vi "DOE Kitchen Agilent.vi"(1 "Flow Rate":dbl, 4 "Water Pressure":dbl, 5 "Data Logger Type":T13=enum."Agilent", 6 "Disable Digital":bool, 7 "Water Temperature":dbl, 8 "error in (no error)":errorcluster, 9 "Test Fixture Hardware":T7={"Power "={"Yokogawa"={"WT210"={"Sample Rate (1: 0.25s)"=1, "A Range (12: 20A)"=11, "V Range (6: 600V)"=4, "Power VISA Yokogawa WT210"=""}, "WT500"={"Power VISA Yokogawa WT500"="", "V Range (8: 1000V)"=6, "I Range (7: 40A)"=7, "Update Rate (3: 500ms)"=2}, "WT310_2"={"Sample Rate (1: 0.25s)"=1, "A Range (12: 20A)"=11, "V Range (6: 600V)"=4, "Power VISA Yokogawa WT310_2"=""}, "WT310_3"={"Sample Rate (1: 0.25s)"=1, "A Range (12: 20A)"=11, "V Range (6: 600V)"=4, "Power VISA Yokogawa WT310_3"=""}}, "Aplus"={"Aplus IP Address"="192.168.1.101", "Remote Port"=502, "Instrument"="APLUS", "Instr Driver Revision"="1.03.0053"}, "Power Limits"={"Crest Factor"={"Upper Limit"=1.49, "Lower Limit"=1.34}, "Harmonic Content"={"Uthd"=2.0}, "Voltage"={"% Error"=2.0}, "Stability"={"<1 Watt "={"Wattage"=1.0, "Slope (mW/H)"=10.0}, ">1 Watt"={"1%Power/Hour"=1.0}}}, "Nominal Voltage"=120, "Time Limit (s)"=10800.0, "Power Variation Limit (%)"=50.0, "Power Supply"={"Chroma 61605"="CHROMA", "Use Chroma?"=FALSE}}, "Weight Scale"={"Com Options"={"IND560Scale VISA"="MW100", "IP Address"="", "Remote Port"=502, "Setra Scale VISA"="MW100", "GSE 350"="GSE350"}, "Select Scale"=""}, "Flow Rates"={"Laurel Cold IP Address"="", "Laurel Hot IP Address"="", "Hot Water Laurel VISA"="LaurelMeter_Hot", "Cold Water Laurel VISA"="LaurelMeter_Cold", "Remote Port"=0, "Laurel Communication Type"="", "Meters To Collect (Hot Cold)"="", "HOT Laurel Reference"=refnum, "COLD Laurel Reference"=refnum}, "Analog Data"={"Agilent"={"Agilent 34972_1"="34972A_1", "Agilent 34972_2"="34972A_2", "Agilent 34972_3"="34972A_3", "Agilent 34972_4"="34972A_3", "Agilent 34972_5"="34972A_3", "Agilent 34972_6"="34972A_3", "Agilent Gain"=0.0, "TC Type (K,J,T)"="", "Instrument IDN?"="", "TC Channels-List"="", "Analog Channels-List"="", "Agilent Cluster Array"=[], "TC Channels-List 2"="", "Analog Channels-List 2"=""}, "Yokogawa"={"MW100"="MW100", "Intellifaucet"=FALSE}, "Select Analog"="", "TC Coefficients"={"TC Coefficients 1"=[], "TC Coefficients 2"=[], "TC Coefficients 3"=[], "TC Coefficients 4"=[], "TC Coefficients 5"=[], "TC Coefficients 6"=[], "TC Coefficients 7"=[]}, "NI Tasks (Dryer DOE)"=["TC Temps-Module 1", "TC Temps-Module 2", "TC Temps-Module 3", "TC Temps-Module 4", "TC Temps-Module 5", "Gas and Temp-Module 6", "AC_DC Events-Module 7"], "Laurel Analog"={"Laurel IP (Water Temp)"="", "Laurel IP (Pressure)"=""}}, "ITHX-Temp Humidity"={"IP Address 1"="", "Remote Port"=0, "IP Address 2"="", "IP Address 3"=""}, "Gas Meter COM Ports"={"Gas Meter 1"="COM3", "Gas Meter 2"="COM4", "Gas Meter 3"="COM5", "Gas Meter 4"="COM6", "Gas Meter 5"="COM7", "Gas Meter 6"="COM8"}, "Barometric Pressure"={"HEISE 901A"="HEISE", "Use Barometer?"=FALSE}} {"Power"."Yokogawa"."WT310_3"."V Range (6: 600V)" items=["Auto", "15V", "30V", "60V", "150V", "300V", "600V"]; "Power"."Yokogawa"."WT310_3"."A Range (12: 20A)" items=["Auto", "5mA", "10mA", "20mA", "50mA", "100mA", "200mA", "0.5A", "1A", "2A", "5A", "10A", "20A", "50mV", "100mV", "200mV", "2.5V", "5V", "10V"]; "Power"."Yokogawa"."WT310_3"."Sample Rate (1: 0.25s)" items=["0.1s", "0.25s", "0.5s", "1s", "2s", "5s"]; "Power"."Yokogawa"."WT310_2"."V Range (6: 600V)" items=["Auto", "15V", "30V", "60V", "150V", "300V", "600V"]; "Power"."Yokogawa"."WT310_2"."A Range (12: 20A)" items=["Auto", "5mA", "10mA", "20mA", "50mA", "100mA", "200mA", "0.5A", "1A", "2A", "5A", "10A", "20A", "50mV", "100mV", "200mV", "2.5V", "5V", "10V"]; "Power"."Yokogawa"."WT310_2"."Sample Rate (1: 0.25s)" items=["0.1s", "0.25s", "0.5s", "1s", "2s", "5s"]; "Power"."Yokogawa"."WT500"."Update Rate (3: 500ms)" items=["-", "100ms", "200ms", "500ms", "1s", "2s", "5s"]; "Power"."Yokogawa"."WT500"."I Range (7: 40A)" items=["AUTO", "500 mA", "1 A", "2 A", "5 A", "10 A", "20 A", "40 A", "S-AUTO", "50 mV", "100 mV", "200 mV", "500 mV", "1 V", "2 V", "5 V", "10 V", "250 mA", "500 mA", "1 A", "2.5 A", "5 A", "10 A", "20 A", "25 mV", "50 mV", "100 mV", "250 mV", "500 mV", "1 V", "2.5 V", "5 V"]; "Power"."Yokogawa"."WT500"."V Range (8: 1000V)" items=["AUTO", "15", "30", "60", "100", "150", "300", "600", "1000", "7.5", "15", "30", "50", "75", "150", "300", "500"]; "Power"."Yokogawa"."WT210"."V Range (6: 600V)" items=["Auto", "15V", "30V", "60V", "150V", "300V", "600V"]; "Power"."Yokogawa"."WT210"."A Range (12: 20A)" items=["Auto", "5mA", "10mA", "20mA", "50mA", "100mA", "200mA", "0.5A", "1A", "2A", "5A", "10A", "20A", "50mV", "100mV", "200mV", "2.5V", "5V", "10V"]; "Power"."Yokogawa"."WT210"."Sample Rate (1: 0.25s)" items=["0.1s", "0.25s", "0.5s", "1s", "2s", "5s"]}, 10 "Measurments":T1={"Power Measurements"={"Current (A):Element 1"=0.0, "Current (A):Element 2"=0.0, "Power (W):Sigma"=0.0, "Watt Hours (Wh):Sigma"=0.0, "Voltage (V):Element 2"=0.0, "Voltage (V):Element 1"=0.0, "Current Crest Factor:Element 1"=0.0, "Current Crest Factor:Element 2"=0.0, "Voltage Harmonic (%):Element 1"=0.0, "Voltage Harmonic (%):Element 2"=0.0, "Voltage Crest Factor:Element 1"=0.0, "Voltage Crest Factor:Element 2"=0.0, "Time:Element 1"=0.0, "Frequency (Hz):Element 1"=0.0, "Apparent Power (VA):Element 1"=0.0, "Apparent Power (VA):Element 2"=0.0, "Power Factor:Element 1"=0.0, "Power Factor:Element 2"=0.0, "Max Watt Hours"=0.0, "Voltage (V):Element 2 Avg"=0.0, "Voltage (V):Element 1 Avg"=0.0}, "Standby Power"={"Standby Power Spreadsheet"=[], "Standby Power - Pia (Watts)"=0.0, "Off Mode Power - Poff (Watts)"=0.0, "Sia hr/yr"=8620.0, "Soff hr/yr"=0.0, "Yearly Energy Etso kWh/yr"=0.0, "Maximum Power (Watts)"=0.0, "Power Variation (%)"=0.0, "Slope (mW/hr)"=0.0, "Final Harmonics-U1 (%)"="", "Final Harmonics-U2 (%)"="", "Energy (Wh)"=0.0}, "Washer"={"Washer String Data"=[], "Analog Scale Weight (lbs)"=0.0}, "Dishwasher"={"Drain Solonoid Event"=0, "Pump Event"=0, "Water Valve Event"=0, "Heater Event"=0, "Motor Event"=0, "Turbidity Sensor"=0.0, "Spare 2"=0.0, "Spare 3"=0.0, "Spare 4"=0.0, "Spare 5"=0.0, "Thermocouple 1"=0.0, "Thermocouple 2"=0.0, "Thermocouple 3"=0.0, "Thermocouple 4"=0.0, "Thermocouple 5"=0.0, "Thermocouple 6"=0.0, "Spare 1"=0.0, "Dishwasher String Data"=[]}, "Washer HCC"={"Chan 101"=0.0, "Chan 102"=0.0, "Chan 103"=0.0, "Chan 104"=0.0, "Chan 105"=0.0, "Chan 106"=0.0, "Chan 107"=0.0, "Chan 108"=0.0, "Chan 109"=0.0, "Chan 110"=0.0, "Chan 111"=0.0, "Chan 112"=0.0, "Chan 113"=0.0, "Chan 114"=0.0, "Chan 115"=0.0, "Chan 116"=0.0, "Chan 117"=0.0, "Chan 118"=0.0, "Chan 119"=0.0, "Chan 120"=0.0, "Chan 201"=0.0, "Chan 202"=0.0, "Chan 203"=0.0, "Chan 204"=0.0, "Chan 205"=0.0, "Chan 206"=0.0, "Chan 207"=0.0, "Chan 208"=0.0, "Chan 209"=0.0, "Chan 210"=0.0, "Chan 211"=0.0, "Chan 212"=0.0, "Chan 213"=0.0, "Chan 214"=0.0, "Chan 215"=0.0, "Chan 216"=0.0, "Chan 217"=0.0, "Chan 218"=0.0, "Chan 219"=0.0, "Chan 220"=0.0, "Chan 301"=0.0, "Chan 302"=0.0, "Chan 303"=0.0, "Chan 304"=0.0, "Chan 305"=0.0, "Chan 306"=0.0, "Chan 307"=0.0, "Chan 308"=0.0, "Chan 309"=0.0, "Chan 310"=0.0, "Chan 311"=0.0, "Chan 312"=0.0, "Chan 313"=0.0, "Chan 314"=0.0, "Chan 315"=0.0, "Chan 316"=0.0, "Chan 317"=0.0, "Chan 318"=0.0, "Chan 319"=0.0, "Chan 320"=0.0}, "Barometric Pressure"={"Barometric Pressure (in. Hg)"=0.0}, "Ambient Conditions"={"Ambient Temperature  1 (°F)"=0.0, "Ambient Temperature 2 (°F)"=0.0, "Ambient Temperature 3 (°F)"=0.0, "Ambient Humidity 1 (%)"=0.0, "Ambient Humidity 2 (%)"=0.0, "Ambient Humidity 3 (%)"=0.0, "Ambient Dewpoint  1 (°F)"=0.0, "Ambient Dewpoint 2 (°F)"=0.0, "Ambient Dewpoint 3 (°F)"=0.0}, "Weight Scale"={"Gross Weigth (lbs)"=0.0, "Net Weight (lbs)"=0.0, "Final Weight (lbs)"=""}, "Water Measurements"={"Hot Water Pressure (psi)"=0.0, "Hot Water Pressure Max (psi)"=0.0, "Hot Water Temperature (°F)"=0.0, "Cold Water Pressure (psi)"=0.0, "Cold Water Pressure Max (psi)"=0.0, "Hot Water Temperature Max (°F)"=0.0, "Cold Water Temperature (°F)"=0.0, "Cold Water Temperature Max (°F)"=0.0, "Hot Water Total (Gal)"=0.0, "Hot Water Rate (GPM)"=0.0, "Cold Water Total (Gal)"=0.0, "Cold Water Rate (GPM)"=0.0, "Cold Water Total During Wash (Gal)"=0.0, "Hot Water Total During Wash (Gal)"=0.0, "Rinse Cold (Gal)"=0.0, "Rinse Hot (Gal)"=0.0, "Hot Water Pressure Min (psi)"=0.0, "Hot Water Temperature Min (°F)"=0.0, "Cold Water Pressure Min (psi)"=0.0, "Cold Water Temperature Min (°F)"=0.0}, "Gas Data"={"Meter Type (Gas)"="", "Meter ID"=enum."Disabled", "Heating Value (BTU/ft³)"=0.0, "Ft³ / Hr (SCFH)"=0.0, "15 Second Average (BTU/HR)"=0.0, "30 Second Average (BTU/HR)"=0.0, "SLPM (Mass Flow)"=0.0, "LPM (Vol. Flow)"=0.0, "Gas Temperature (°F)"=0.0, "Gas Pressure (PSIA)"=0.0, "Tot.Flow (Liters)"=0.0}} {"Power Measurements"."Voltage (V):Element 1 Avg" format="%.3g"; "Power Measurements"."Voltage (V):Element 2 Avg" format="%.3g"; "Power Measurements"."Max Watt Hours" format="%.3g"; "Power Measurements"."Power Factor:Element 2" format="%.3g"; "Power Measurements"."Power Factor:Element 1" format="%.3g"; "Power Measurements"."Apparent Power (VA):Element 2" format="%.3g"; "Power Measurements"."Apparent Power (VA):Element 1" format="%.3g"; "Power Measurements"."Frequency (Hz):Element 1" format="%.3g"; "Power Measurements"."Time:Element 1" format="%.3g"; "Power Measurements"."Voltage Crest Factor:Element 2" format="%.3g"; "Power Measurements"."Voltage Crest Factor:Element 1" format="%.3g"; "Power Measurements"."Voltage Harmonic (%):Element 2" format="%.3g"; "Power Measurements"."Voltage Harmonic (%):Element 1" format="%.3g"; "Power Measurements"."Current Crest Factor:Element 2" format="%.3g"; "Power Measurements"."Current Crest Factor:Element 1" format="%.3g"; "Power Measurements"."Voltage (V):Element 1" format="%.3g"; "Power Measurements"."Voltage (V):Element 2" format="%.3g"; "Power Measurements"."Watt Hours (Wh):Sigma" format="%.3f"; "Power Measurements"."Power (W):Sigma" format="%.3g"; "Power Measurements"."Current (A):Element 2" format="%.3g"; "Power Measurements"."Current (A):Element 1" format="%.3g"}, 11 "VISA Resource Name":refnum<visa-resource-name>) -> (0 "error out":errorcluster, 2 "Measurments Output":T1={"Power Measurements"={"Current (A):Element 1"=0.0, "Current (A):Element 2"=0.0, "Power (W):Sigma"=0.0, "Watt Hours (Wh):Sigma"=0.0, "Voltage (V):Element 2"=0.0, "Voltage (V):Element 1"=0.0, "Current Crest Factor:Element 1"=0.0, "Current Crest Factor:Element 2"=0.0, "Voltage Harmonic (%):Element 1"=0.0, "Voltage Harmonic (%):Element 2"=0.0, "Voltage Crest Factor:Element 1"=0.0, "Voltage Crest Factor:Element 2"=0.0, "Time:Element 1"=0.0, "Frequency (Hz):Element 1"=0.0, "Apparent Power (VA):Element 1"=0.0, "Apparent Power (VA):Element 2"=0.0, "Power Factor:Element 1"=0.0, "Power Factor:Element 2"=0.0, "Max Watt Hours"=0.0, "Voltage (V):Element 2 Avg"=0.0, "Voltage (V):Element 1 Avg"=0.0}, "Standby Power"={"Standby Power Spreadsheet"=[], "Standby Power - Pia (Watts)"=0.0, "Off Mode Power - Poff (Watts)"=0.0, "Sia hr/yr"=8620.0, "Soff hr/yr"=0.0, "Yearly Energy Etso kWh/yr"=0.0, "Maximum Power (Watts)"=0.0, "Power Variation (%)"=0.0, "Slope (mW/hr)"=0.0, "Final Harmonics-U1 (%)"="", "Final Harmonics-U2 (%)"="", "Energy (Wh)"=0.0}, "Washer"={"Washer String Data"=[], "Analog Scale Weight (lbs)"=0.0}, "Dishwasher"={"Drain Solonoid Event"=0, "Pump Event"=0, "Water Valve Event"=0, "Heater Event"=0, "Motor Event"=0, "Turbidity Sensor"=0.0, "Spare 2"=0.0, "Spare 3"=0.0, "Spare 4"=0.0, "Spare 5"=0.0, "Thermocouple 1"=0.0, "Thermocouple 2"=0.0, "Thermocouple 3"=0.0, "Thermocouple 4"=0.0, "Thermocouple 5"=0.0, "Thermocouple 6"=0.0, "Spare 1"=0.0, "Dishwasher String Data"=[]}, "Washer HCC"={"Chan 101"=0.0, "Chan 102"=0.0, "Chan 103"=0.0, "Chan 104"=0.0, "Chan 105"=0.0, "Chan 106"=0.0, "Chan 107"=0.0, "Chan 108"=0.0, "Chan 109"=0.0, "Chan 110"=0.0, "Chan 111"=0.0, "Chan 112"=0.0, "Chan 113"=0.0, "Chan 114"=0.0, "Chan 115"=0.0, "Chan 116"=0.0, "Chan 117"=0.0, "Chan 118"=0.0, "Chan 119"=0.0, "Chan 120"=0.0, "Chan 201"=0.0, "Chan 202"=0.0, "Chan 203"=0.0, "Chan 204"=0.0, "Chan 205"=0.0, "Chan 206"=0.0, "Chan 207"=0.0, "Chan 208"=0.0, "Chan 209"=0.0, "Chan 210"=0.0, "Chan 211"=0.0, "Chan 212"=0.0, "Chan 213"=0.0, "Chan 214"=0.0, "Chan 215"=0.0, "Chan 216"=0.0, "Chan 217"=0.0, "Chan 218"=0.0, "Chan 219"=0.0, "Chan 220"=0.0, "Chan 301"=0.0, "Chan 302"=0.0, "Chan 303"=0.0, "Chan 304"=0.0, "Chan 305"=0.0, "Chan 306"=0.0, "Chan 307"=0.0, "Chan 308"=0.0, "Chan 309"=0.0, "Chan 310"=0.0, "Chan 311"=0.0, "Chan 312"=0.0, "Chan 313"=0.0, "Chan 314"=0.0, "Chan 315"=0.0, "Chan 316"=0.0, "Chan 317"=0.0, "Chan 318"=0.0, "Chan 319"=0.0, "Chan 320"=0.0}, "Barometric Pressure"={"Barometric Pressure (in. Hg)"=0.0}, "Ambient Conditions"={"Ambient Temperature  1 (°F)"=0.0, "Ambient Temperature 2 (°F)"=0.0, "Ambient Temperature 3 (°F)"=0.0, "Ambient Humidity 1 (%)"=0.0, "Ambient Humidity 2 (%)"=0.0, "Ambient Humidity 3 (%)"=0.0, "Ambient Dewpoint  1 (°F)"=0.0, "Ambient Dewpoint 2 (°F)"=0.0, "Ambient Dewpoint 3 (°F)"=0.0}, "Weight Scale"={"Gross Weigth (lbs)"=0.0, "Net Weight (lbs)"=0.0, "Final Weight (lbs)"=""}, "Water Measurements"={"Hot Water Pressure (psi)"=0.0, "Hot Water Pressure Max (psi)"=0.0, "Hot Water Temperature (°F)"=0.0, "Cold Water Pressure (psi)"=0.0, "Cold Water Pressure Max (psi)"=0.0, "Hot Water Temperature Max (°F)"=0.0, "Cold Water Temperature (°F)"=0.0, "Cold Water Temperature Max (°F)"=0.0, "Hot Water Total (Gal)"=0.0, "Hot Water Rate (GPM)"=0.0, "Cold Water Total (Gal)"=0.0, "Cold Water Rate (GPM)"=0.0, "Cold Water Total During Wash (Gal)"=0.0, "Hot Water Total During Wash (Gal)"=0.0, "Rinse Cold (Gal)"=0.0, "Rinse Hot (Gal)"=0.0, "Hot Water Pressure Min (psi)"=0.0, "Hot Water Temperature Min (°F)"=0.0, "Cold Water Pressure Min (psi)"=0.0, "Cold Water Temperature Min (°F)"=0.0}, "Gas Data"={"Meter Type (Gas)"="", "Meter ID"=enum."Disabled", "Heating Value (BTU/ft³)"=0.0, "Ft³ / Hr (SCFH)"=0.0, "15 Second Average (BTU/HR)"=0.0, "30 Second Average (BTU/HR)"=0.0, "SLPM (Mass Flow)"=0.0, "LPM (Vol. Flow)"=0.0, "Gas Temperature (°F)"=0.0, "Gas Pressure (PSIA)"=0.0, "Tot.Flow (Liters)"=0.0}} {"Power Measurements"."Voltage (V):Element 1 Avg" format="%.3g"; "Power Measurements"."Voltage (V):Element 2 Avg" format="%.3g"; "Power Measurements"."Max Watt Hours" format="%.3g"; "Power Measurements"."Power Factor:Element 2" format="%.3g"; "Power Measurements"."Power Factor:Element 1" format="%.3g"; "Power Measurements"."Apparent Power (VA):Element 2" format="%.3g"; "Power Measurements"."Apparent Power (VA):Element 1" format="%.3g"; "Power Measurements"."Frequency (Hz):Element 1" format="%.3g"; "Power Measurements"."Time:Element 1" format="%.3g"; "Power Measurements"."Voltage Crest Factor:Element 2" format="%.3g"; "Power Measurements"."Voltage Crest Factor:Element 1" format="%.3g"; "Power Measurements"."Voltage Harmonic (%):Element 2" format="%.3g"; "Power Measurements"."Voltage Harmonic (%):Element 1" format="%.3g"; "Power Measurements"."Current Crest Factor:Element 2" format="%.3g"; "Power Measurements"."Current Crest Factor:Element 1" format="%.3g"; "Power Measurements"."Voltage (V):Element 1" format="%.3g"; "Power Measurements"."Voltage (V):Element 2" format="%.3g"; "Power Measurements"."Watt Hours (Wh):Sigma" format="%.3f"; "Power Measurements"."Power (W):Sigma" format="%.3g"; "Power Measurements"."Current (A):Element 2" format="%.3g"; "Power Measurements"."Current (A):Element 1" format="%.3g"}, 3 "Kitchen Analog Data":string[][](array[string]))   [LabVIEW 2018]
uses:
  Type Definitions/DOE Data Logger Type.ctl
  Type Definitions/DOE Test Fixture Hardware.ctl
  Utility/Type Definitions/UTILITY Power Inputs Control.ctl
  Drivers/IND560 Scale Monitor/Type Definitions/IND560 Configuration.ctl
  Hybrid Water Heater/Type Definitions/HEWH Agilent Cluster.ctl
  Utility/Type Definitions/UTILITY TC Coefficients.ctl
  Drivers/Omega FMA-1600A Series Gas Flow Meter/Type Definitions/FMA1600A COM Ports.ctl
  Type Definitions/DOE Front Panel Meters.ctl
  Utility/Type Definitions/UTILITY Power Data.ctl
  Utility/Standby Power/Type Definitions/Standby Power Main Data.ctl
  Drivers/Omega FMA-1600A Series Gas Flow Meter/Type Definitions/FMA1600A Gas Data.ctl
  Drivers/Omega FMA-1600A Series Gas Flow Meter/Type Definitions/FMA1600A Gas Type.ctl
  Range/Type Definitions/RANGE Meter Selector 1-2.ctl
  Drivers/Yokogawa MW100/Type Definitions/YKMW100 DISH Channel Settings.ctl
  Drivers/Agilent 34972/Agilent 34970.lvlib
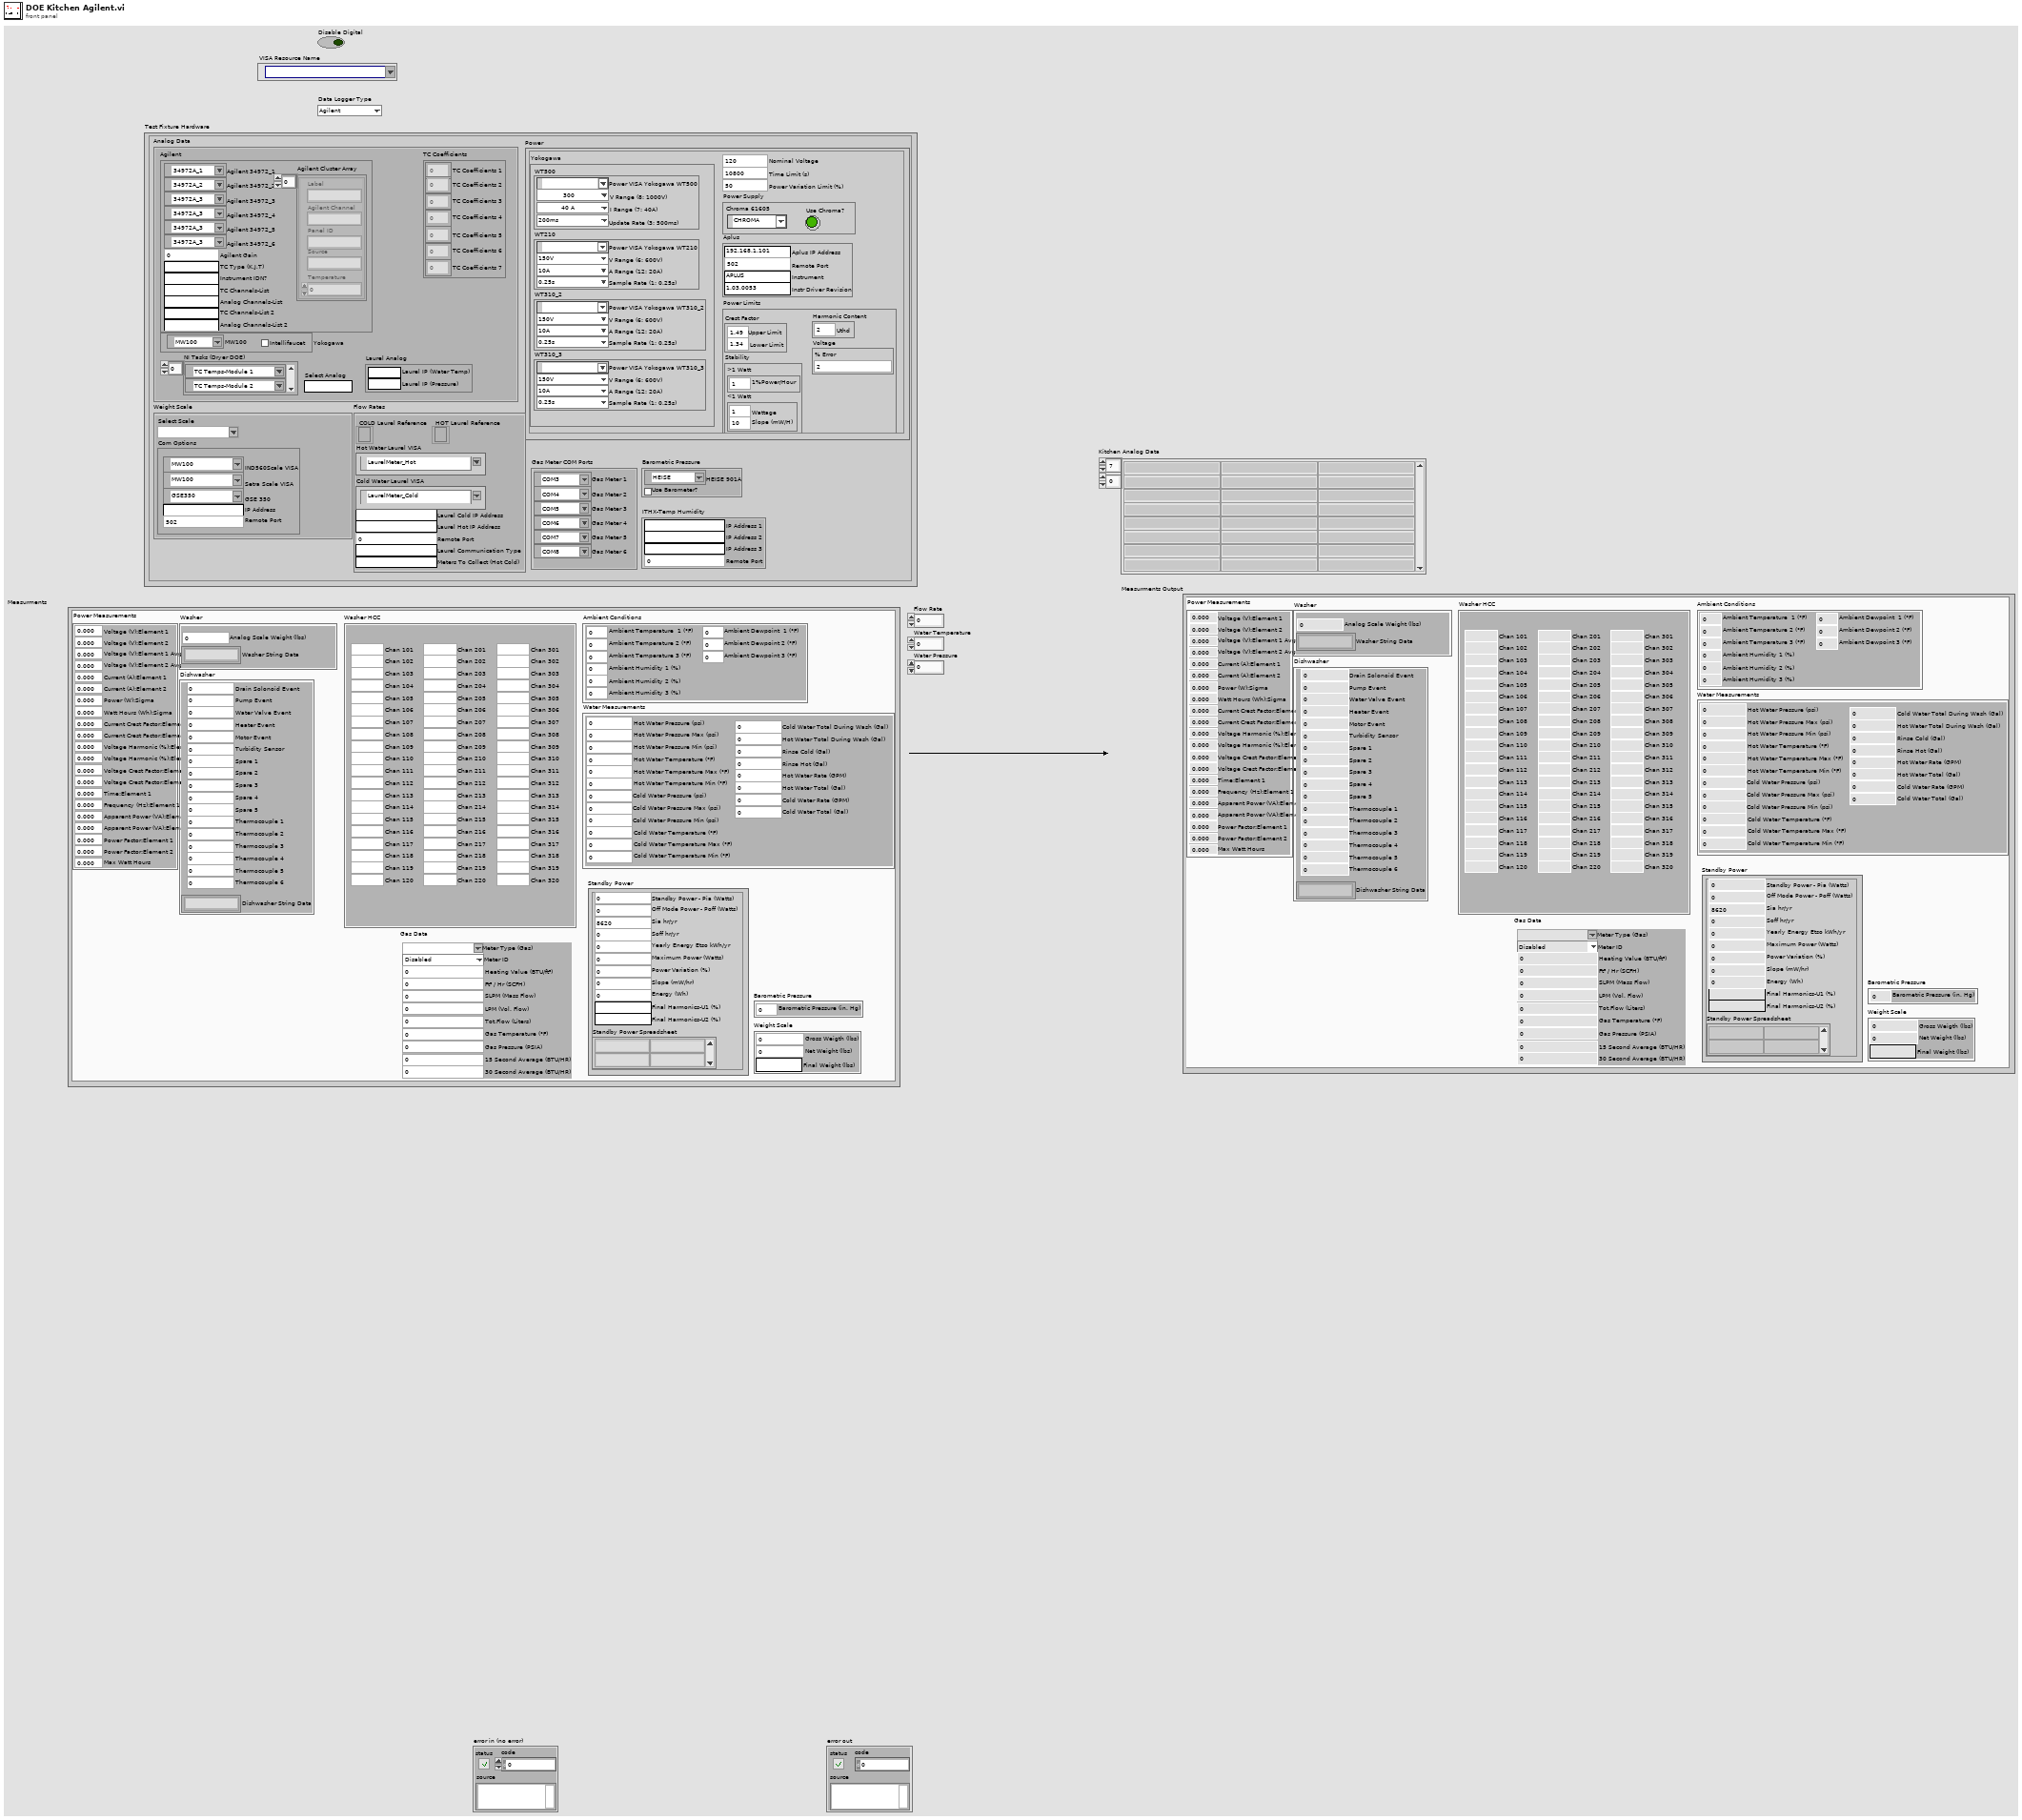
[diagram p1: front panel]
types:
  T1 = typedef "DOE Front Panel Meters.ctl" = cluster{"Power Measurements":T2, "Standby Power":T3, "Washer":cluster{"Washer String Data":string[][], "Analog Scale Weight (lbs)":dbl}, "Dishwasher":cluster{"Drain Solonoid Event":i32, "Pump Event":i32, "Water Valve Event":i32, "Heater Event":i32, "Motor Event":i32, "Turbidity Sensor":dbl, "Spare 2":dbl, "Spare 3":dbl, "Spare 4":dbl, "Spare 5":dbl, "Thermocouple 1":dbl, "Thermocouple 2":dbl, "Thermocouple 3":dbl, "Thermocouple 4":dbl, "Thermocouple 5":dbl, "Thermocouple 6":dbl, "Spare 1":dbl, "Dishwasher String Data":string[][]}, "Washer HCC":cluster{"Chan 101":dbl, "Chan 102":dbl, "Chan 103":dbl, "Chan 104":dbl, "Chan 105":dbl, "Chan 106":dbl, "Chan 107":dbl, "Chan 108":dbl, "Chan 109":dbl, "Chan 110":dbl, "Chan 111":dbl, "Chan 112":dbl, "Chan 113":dbl, "Chan 114":dbl, "Chan 115":dbl, "Chan 116":dbl, "Chan 117":dbl, "Chan 118":dbl, "Chan 119":dbl, "Chan 120":dbl, "Chan 201":dbl, "Chan 202":dbl, "Chan 203":dbl, "Chan 204":dbl, "Chan 205":dbl, "Chan 206":dbl, "Chan 207":dbl, "Chan 208":dbl, "Chan 209":dbl, "Chan 210":dbl, "Chan 211":dbl, "Chan 212":dbl, "Chan 213":dbl, "Chan 214":dbl, "Chan 215":dbl, "Chan 216":dbl, "Chan 217":dbl, "Chan 218":dbl, "Chan 219":dbl, "Chan 220":dbl, "Chan 301":dbl, "Chan 302":dbl, "Chan 303":dbl, "Chan 304":dbl, "Chan 305":dbl, "Chan 306":dbl, "Chan 307":dbl, "Chan 308":dbl, "Chan 309":dbl, "Chan 310":dbl, "Chan 311":dbl, "Chan 312":dbl, "Chan 313":dbl, "Chan 314":dbl, "Chan 315":dbl, "Chan 316":dbl, "Chan 317":dbl, "Chan 318":dbl, "Chan 319":dbl, "Chan 320":dbl}, "Barometric Pressure":cluster{"Barometric Pressure (in. Hg)":dbl}, "Ambient Conditions":cluster{"Ambient Temperature  1 (°F)":dbl, "Ambient Temperature 2 (°F)":dbl, "Ambient Temperature 3 (°F)":dbl, "Ambient Humidity 1 (%)":dbl, "Ambient Humidity 2 (%)":dbl, "Ambient Humidity 3 (%)":dbl, "Ambient Dewpoint  1 (°F)":dbl, "Ambient Dewpoint 2 (°F)":dbl, "Ambient Dewpoint 3 (°F)":dbl}, "Weight Scale":cluster{"Gross Weigth (lbs)":dbl, "Net Weight (lbs)":dbl, "Final Weight (lbs)":string}, "Water Measurements":cluster{"Hot Water Pressure (psi)":dbl, "Hot Water Pressure Max (psi)":dbl, "Hot Water Temperature (°F)":dbl, "Cold Water Pressure (psi)":dbl, "Cold Water Pressure Max (psi)":dbl, "Hot Water Temperature Max (°F)":dbl, "Cold Water Temperature (°F)":dbl, "Cold Water Temperature Max (°F)":dbl, "Hot Water Total (Gal)":dbl, "Hot Water Rate (GPM)":dbl, "Cold Water Total (Gal)":dbl, "Cold Water Rate (GPM)":dbl, "Cold Water Total During Wash (Gal)":dbl, "Hot Water Total During Wash (Gal)":dbl, "Rinse Cold (Gal)":dbl, "Rinse Hot (Gal)":dbl, "Hot Water Pressure Min (psi)":dbl, "Hot Water Temperature Min (°F)":dbl, "Cold Water Pressure Min (psi)":dbl, "Cold Water Temperature Min (°F)":dbl}, "Gas Data":T4}
  T2 = typedef "UTILITY Power Data.ctl" = cluster{"Current (A):Element 1":dbl, "Current (A):Element 2":dbl, "Power (W):Sigma":dbl, "Watt Hours (Wh):Sigma":dbl, "Voltage (V):Element 2":dbl, "Voltage (V):Element 1":dbl, "Current Crest Factor:Element 1":dbl, "Current Crest Factor:Element 2":dbl, "Voltage Harmonic (%):Element 1":dbl, "Voltage Harmonic (%):Element 2":dbl, "Voltage Crest Factor:Element 1":dbl, "Voltage Crest Factor:Element 2":dbl, "Time:Element 1":dbl, "Frequency (Hz):Element 1":dbl, "Apparent Power (VA):Element 1":dbl, "Apparent Power (VA):Element 2":dbl, "Power Factor:Element 1":dbl, "Power Factor:Element 2":dbl, "Max Watt Hours":dbl, "Voltage (V):Element 2 Avg":dbl, "Voltage (V):Element 1 Avg":dbl}
  T3 = typedef "Standby Power Main Data.ctl" = cluster{"Standby Power Spreadsheet":string[][], "Standby Power - Pia (Watts)":dbl, "Off Mode Power - Poff (Watts)":dbl, "Sia hr/yr":dbl, "Soff hr/yr":dbl, "Yearly Energy Etso kWh/yr":dbl, "Maximum Power (Watts)":dbl, "Power Variation (%)":dbl, "Slope (mW/hr)":dbl, "Final Harmonics-U1 (%)":string, "Final Harmonics-U2 (%)":string, "Energy (Wh)":dbl}
  T4 = typedef "FMA1600A Gas Data.ctl" = cluster{"Meter Type (Gas)":T5, "Meter ID":T6, "Heating Value (BTU/ft³)":dbl, "Ft³ / Hr (SCFH)":dbl, "15 Second Average (BTU/HR)":dbl, "30 Second Average (BTU/HR)":dbl, "SLPM (Mass Flow)":dbl, "LPM (Vol. Flow)":dbl, "Gas Temperature (°F)":dbl, "Gas Pressure (PSIA)":dbl, "Tot.Flow (Liters)":dbl}
  T5 = typedef "FMA1600A Gas Type.ctl" = string
  T6 = typedef "RANGE Meter Selector 1-2.ctl" = enum16{"Disabled", "Meter 1", "Meter 2", "Auto"}
  T7 = typedef "DOE Test Fixture Hardware.ctl" = cluster{"Power ":T8, "Weight Scale":cluster{"Com Options":T9, "Select Scale":string}, "Flow Rates":cluster{"Laurel Cold IP Address":string, "Laurel Hot IP Address":string, "Hot Water Laurel VISA":refnum<visa-resource-name>, "Cold Water Laurel VISA":refnum<visa-resource-name>, "Remote Port":u16, "Laurel Communication Type":string, "Meters To Collect (Hot Cold)":string, "HOT Laurel Reference":refnum<k5>, "COLD Laurel Reference":refnum<k5>}, "Analog Data":cluster{"Agilent":cluster{"Agilent 34972_1":refnum<visa-resource-name>, "Agilent 34972_2":refnum<visa-resource-name>, "Agilent 34972_3":refnum<visa-resource-name>, "Agilent 34972_4":refnum<visa-resource-name>, "Agilent 34972_5":refnum<visa-resource-name>, "Agilent 34972_6":refnum<visa-resource-name>, "Agilent Gain":dbl, "TC Type (K,J,T)":string, "Instrument IDN?":string, "TC Channels-List":string, "Analog Channels-List":string, "Agilent Cluster Array":T10[], "TC Channels-List 2":string, "Analog Channels-List 2":string}, "Yokogawa":cluster{"MW100":refnum<visa-resource-name>, "Intellifaucet":bool}, "Select Analog":string, "TC Coefficients":T11, "NI Tasks (Dryer DOE)":refnum<k21>[], "Laurel Analog":cluster{"Laurel IP (Water Temp)":string, "Laurel IP (Pressure)":string}}, "ITHX-Temp Humidity":cluster{"IP Address 1":string, "Remote Port":u16, "IP Address 2":string, "IP Address 3":string}, "Gas Meter COM Ports":T12, "Barometric Pressure":cluster{"HEISE 901A":refnum<visa-resource-name>, "Use Barometer?":bool}}
  T8 = typedef "UTILITY Power Inputs Control.ctl" = cluster{"Yokogawa":cluster{"WT210":cluster{"Sample Rate (1: 0.25s)":i32, "A Range (12: 20A)":i32, "V Range (6: 600V)":i32, "Power VISA Yokogawa WT210":refnum<visa-resource-name>}, "WT500":cluster{"Power VISA Yokogawa WT500":refnum<visa-resource-name>, "V Range (8: 1000V)":i32, "I Range (7: 40A)":i32, "Update Rate (3: 500ms)":i32}, "WT310_2":cluster{"Sample Rate (1: 0.25s)":i32, "A Range (12: 20A)":i32, "V Range (6: 600V)":i32, "Power VISA Yokogawa WT310_2":refnum<visa-resource-name>}, "WT310_3":cluster{"Sample Rate (1: 0.25s)":i32, "A Range (12: 20A)":i32, "V Range (6: 600V)":i32, "Power VISA Yokogawa WT310_3":refnum<visa-resource-name>}}, "Aplus":cluster{"Aplus IP Address":string, "Remote Port":i32, "Instrument":string, "Instr Driver Revision":string}, "Power Limits":cluster{"Crest Factor":cluster{"Upper Limit":dbl, "Lower Limit":dbl}, "Harmonic Content":cluster{"Uthd":dbl}, "Voltage":cluster{"% Error":dbl}, "Stability":cluster{"<1 Watt ":cluster{"Wattage":dbl, "Slope (mW/H)":dbl}, ">1 Watt":cluster{"1%Power/Hour":dbl}}}, "Nominal Voltage":i32, "Time Limit (s)":dbl, "Power Variation Limit (%)":dbl, "Power Supply":cluster{"Chroma 61605":refnum<visa-resource-name>, "Use Chroma?":bool}}
  T9 = typedef "IND560 Configuration.ctl" = cluster{"IND560Scale VISA":refnum<visa-resource-name>, "IP Address":string, "Remote Port":u16, "Setra Scale VISA":refnum<visa-resource-name>, "GSE 350":refnum<visa-resource-name>}
  T10 = typedef "HEWH Agilent Cluster.ctl" = cluster{"Label":string, "Agilent Channel":string, "Panel ID":string, "Source":string, "Temperature":dbl}
  T11 = typedef "UTILITY TC Coefficients.ctl" = cluster{"TC Coefficients 1":dbl[], "TC Coefficients 2":dbl[], "TC Coefficients 3":dbl[], "TC Coefficients 4":dbl[], "TC Coefficients 5":dbl[], "TC Coefficients 6":dbl[], "TC Coefficients 7":dbl[]}
  T12 = typedef "FMA1600A COM Ports.ctl" = cluster{"Gas Meter 1":refnum<visa-resource-name>, "Gas Meter 2":refnum<visa-resource-name>, "Gas Meter 3":refnum<visa-resource-name>, "Gas Meter 4":refnum<visa-resource-name>, "Gas Meter 5":refnum<visa-resource-name>, "Gas Meter 6":refnum<visa-resource-name>}
  T13 = typedef "DOE Data Logger Type.ctl" = enum16{"MW100", "Agilent", "Agilent_Laurel_DC_Clamp"}
  T14 = typedef "YKMW100 DISH Channel Settings.ctl" = u32
  T15 = typedef "DOE Kitchen Control.ctl" = cluster{"Drain_Event":i16, "Pump Event":i16, "Water Valve Event":i16, "Heater Event":i16, "Extra":i16, "Turbidity Sensor":dbl, "Thermocouple 1":dbl, "Thermocouple 2":dbl, "Thermocouple 3":dbl, "Thermocouple 4":dbl, "Thermocouple 5":dbl, "Thermocouple 6":dbl, "Water Temperature":dbl, "Water Pressure":dbl, "Event Current 1":dbl, "Event Current 2":dbl, "Event Current 3":dbl, "Event Current 4":dbl, "Event Current 5":dbl, "Thermocouple 7":dbl}
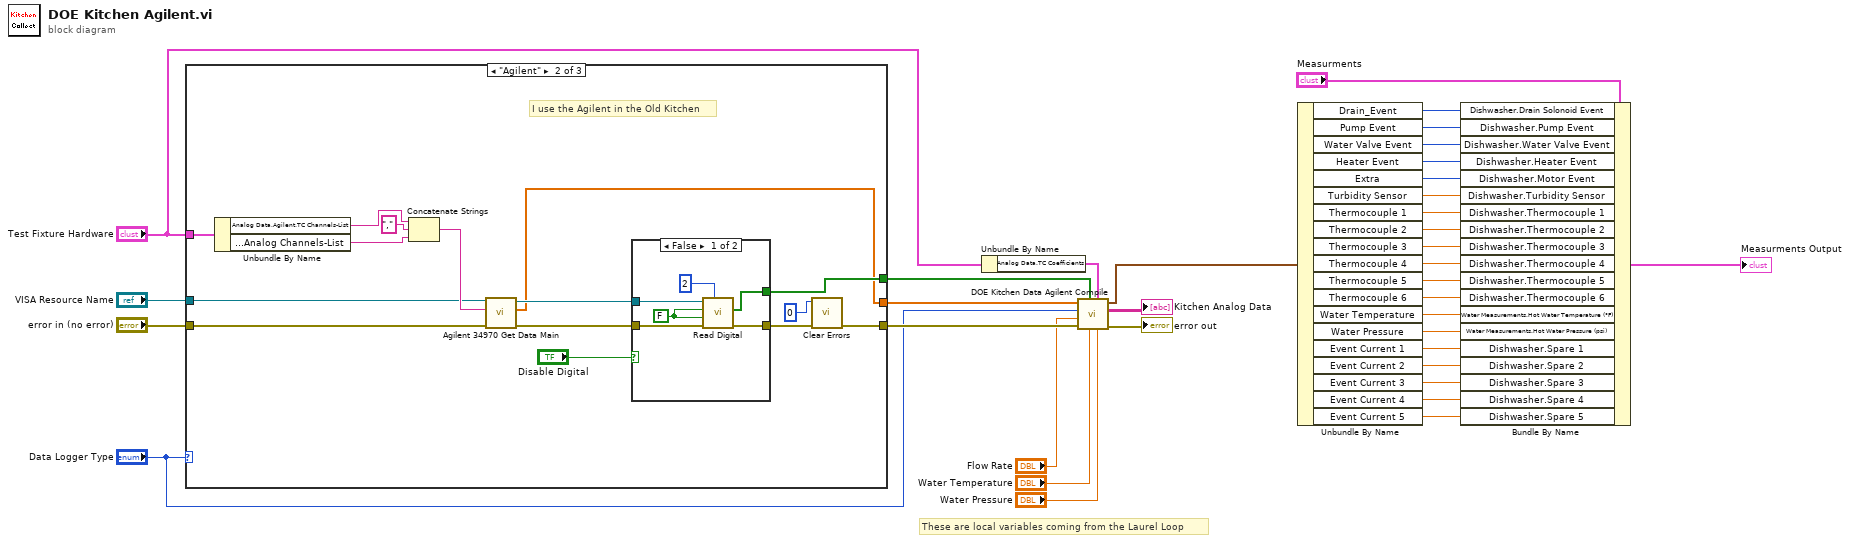
[diagram p0: block diagram]
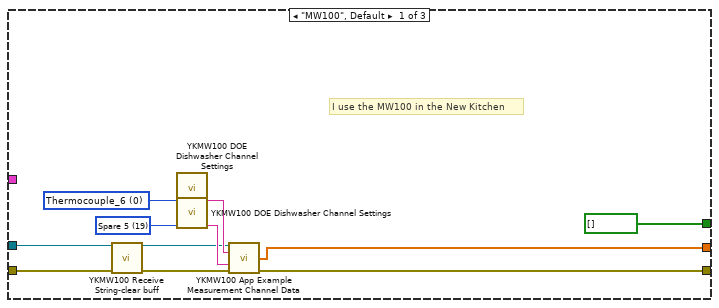
[diagram p2: hidden frame]
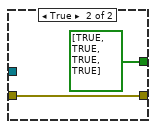
[diagram p3: hidden frame]
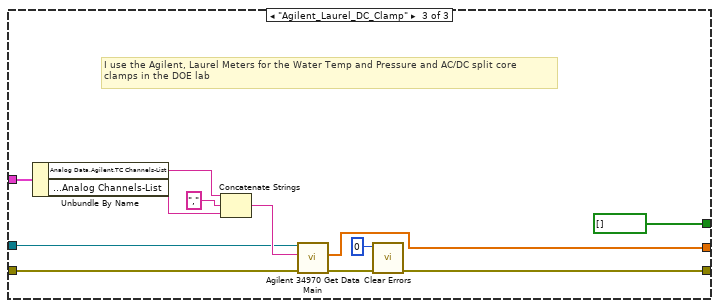
[diagram p4: hidden frame]
diagram:
  # "These are local variables coming from the Laurel Loop"
  n1 = case shown="\"Agilent\"" "Data Logger Type" {
    tunnel: "error in (no error)" -> [w40 w54 w77]
    tunnel: "VISA Resource Name" -> [w39 w52 w76]
    tunnel: [w37 w47 w71] -> w12
    tunnel: "Test Fixture Hardware" -> [_ w60 w75]
    tunnel: [w38 w48 w72] -> w11
    tunnel: [bool[] [] ("Digital Value") w49 bool[] [] ("Digital Value")] -> w4
    frame "MW100", Default {
      w41 = T14 19 items=["Thermocouple_6", "Water Temperature", "Spare 1", "Water_Pressure", "Unit Weight", "Thermocouple 1", "Thermocouple 2", "Thermocouple 3", "Thermocouple 4", "Thermocouple 5", "Drain Event", "Pump Event", "Water Valve Event", "Heater Event", "Motor Event", "Turbidity Sensor", "Spare 2", "Spare 3", "Spare 4", "Spare 5"] ("Channel_Enum")
      w42 = T14 0 items=["Thermocouple_6", "Water Temperature", "Spare 1", "Water_Pressure", "Unit Weight", "Thermocouple 1", "Thermocouple 2", "Thermocouple 3", "Thermocouple 4", "Thermocouple 5", "Drain Event", "Pump Event", "Water Valve Event", "Heater Event", "Motor Event", "Turbidity Sensor", "Spare 2", "Spare 3", "Spare 4", "Spare 5"] ("Channel_Enum")
      # "I use the MW100 in the New Kitchen"
      n2 = call "YKMW100 Receive String-clear buff.vi"("VISA session"=w39, "error in (no error)"=w40) -> ("dup VISA session"=w43:refnum<visa-resource-name>, "error out"=w44:errorcluster)  [unwired: 11 in, 1 out]
      n3 = call "YKMW100 DOE Dishwasher Channel Settings.vi"("Channel_Enum"=w42) -> ("Channel String"=w46:string)  [unwired: 10 in]
      n4 = call "YKMW100 DOE Dishwasher Channel Settings.vi"("Channel_Enum"=w41) -> ("Channel String"=w45:string)  [unwired: 10 in]
      n5 = call "YKMW100 App Example Measurement Channel Data.vi"("VISA session"=w43, "Start Channel (001)"=w46, "End Channel (001)"=w45, "error in (no error)"=w44) -> ("Data List"=w38:dbl[], "error out"=w37:errorcluster)  [unwired: 4 in, 6 out]
    }
    frame "Agilent" {
      # "I use the Agilent in the Old Kitchen"
      n6 = Unbundle By Name(w60) -> ("Analog Data.Agilent.TC Channels-List"=w59:string, "Analog Data.Agilent.Analog Channels-List"=w58:string)
      n7 = Concatenate Strings(w59, "," ("string"), w58) -> (w55:string)
      n8 = call "Agilent 34970 Get Data Main.vi"("error in (no error)"=w54, "Analog Channels-List"=w55, "VISA Refnum in"=w52) -> ("error out"=w53:errorcluster, "Sorted Data"=w48:dbl[], "VISA Resource Name Out"=w51:refnum<visa-resource-name>)  [unwired: 3 in, 3 out]
      n9 = case shown="False" "Disable Digital" {
        tunnel: [w67 bool[] [TRUE, TRUE, TRUE, TRUE] ("Digital Value")] -> w49
        tunnel: w51 -> [w65 _]
        tunnel: [w63 w69] -> w57
        tunnel: w53 -> [w62 w69]
        frame False {
          w66 = FALSE ("Byte/Word (F:Byte)")
          n10 = call "Read Digital.vi"("Slot Number (1)"=u8 2, "error in (no error)"=w62, "Digital Port (F:1)"=w66, "Byte/Word (F:Byte)"=w66, "VISA Resource Name"=w65) -> ("error out"=w63:errorcluster, "Digital Value"=w67:bool[])  [unwired: 4 in, 1 out]
        }
        frame True {
        }
      }
      n11 = call <vilib>:"Clear Errors.vi"("error in (no error)"=w57, "specific error code to clear (0: all)"=0) -> ("error out"=w47:errorcluster)  [unwired: 4 in, 1 out]
    }
    frame "Agilent_Laurel_DC_Clamp" {
      # "I use the Agilent, Laurel Meters for the Water Temp and Pressure and AC/DC split core\nclamps in the DOE lab"
      n12 = Unbundle By Name(w75) -> ("Analog Data.Agilent.TC Channels-List"=w80:string, "Analog Data.Agilent.Analog Channels-List"=w79:string)
      n13 = Concatenate Strings(w80, "," ("string"), w79) -> (w78:string)
      n14 = call "Agilent 34970 Get Data Main.vi"("error in (no error)"=w77, "Analog Channels-List"=w78, "VISA Refnum in"=w76) -> ("error out"=w74:errorcluster, "Sorted Data"=w72:dbl[])  [unwired: 3 in, 4 out]
      n15 = call <vilib>:"Clear Errors.vi"("error in (no error)"=w74, "specific error code to clear (0: all)"=0) -> ("error out"=w71:errorcluster)  [unwired: 4 in, 1 out]
    }
  }
  n16 = Unbundle By Name("Test Fixture Hardware") -> ("Analog Data.TC Coefficients"=w2:T11)
  n17 = call "DOE Kitchen Data Agilent Compile.vi"("Water Pressure"="Water Pressure", "TC Coefficients"=w2, "Water Temperature"="Water Temperature", "Agilent Digital Events"=w4, "Error In"=w12, "Flow Rate"="Flow Rate", "Data Logger Type"="Data Logger Type", "Data Input"=w11) -> ("Error Out"=→"error out":errorcluster, "Kitchen Analog Data"=→"Kitchen Analog Data":string[][], "Kitchen Cluster"=w7:T15)  [unwired: 1 in]
  n18 = Unbundle By Name(w7) -> ("Drain_Event"=w16:i16, "Pump Event"=w17:i16, "Water Valve Event"=w18:i16, "Heater Event"=w19:i16, "Extra"=w20:i16, "Turbidity Sensor"=w21:dbl, "Thermocouple 1"=w22:dbl, "Thermocouple 2"=w23:dbl, "Thermocouple 3"=w24:dbl, "Thermocouple 4"=w25:dbl, "Thermocouple 5"=w26:dbl, "Thermocouple 6"=w27:dbl, "Water Temperature"=w28:dbl, "Water Pressure"=w29:dbl, "Event Current 1"=w30:dbl, "Event Current 2"=w31:dbl, "Event Current 3"=w32:dbl, "Event Current 4"=w33:dbl, "Event Current 5"=w34:dbl)
  n19 = Bundle By Name(cluster="Measurments", "Dishwasher.Drain Solonoid Event"=w16, "Dishwasher.Pump Event"=w17, "Dishwasher.Water Valve Event"=w18, "Dishwasher.Heater Event"=w19, "Dishwasher.Motor Event"=w20, "Dishwasher.Turbidity Sensor"=w21, "Dishwasher.Thermocouple 1"=w22, "Dishwasher.Thermocouple 2"=w23, "Dishwasher.Thermocouple 3"=w24, "Dishwasher.Thermocouple 4"=w25, "Dishwasher.Thermocouple 5"=w26, "Dishwasher.Thermocouple 6"=w27, "Water Measurements.Hot Water Temperature (°F)"=w28, "Water Measurements.Hot Water Pressure (psi)"=w29, "Dishwasher.Spare 1"=w30, "Dishwasher.Spare 2"=w31, "Dishwasher.Spare 3"=w32, "Dishwasher.Spare 4"=w33, "Dishwasher.Spare 5"=w34) -> (→"Measurments Output":T1)
